vi "GenerateScanEndPts.vi"(0 "X Start":sgl, 1 "Mode":enum16{"Raster", "Serpentine"}(ring), 2 "Calibration In":cluster{dbl, "MicrostepMode":u32}[](array[cluster]), 5 "X End":sgl=9.0, 7 "Y Start":sgl, 9 "Y End":sgl=10.0, 11 "error in":errorcluster, 12 "Line Count":u64=6, 13 "Pixel Count":u64=6, 14 "EdgePt/nPixelMap":bool) -> (4 "Coordinate Array":sgl[][](array[numeric]), 6 "X Pixel Count":u64, 8 "Step Sizes":sgl[](array[numeric]), 10 "Y Pixel Count":u64, 15 "error out":errorcluster)   [LabVIEW 2020]
panel:
  out "Pixel Map":cluster{dbl[], dbl[]}(graph)
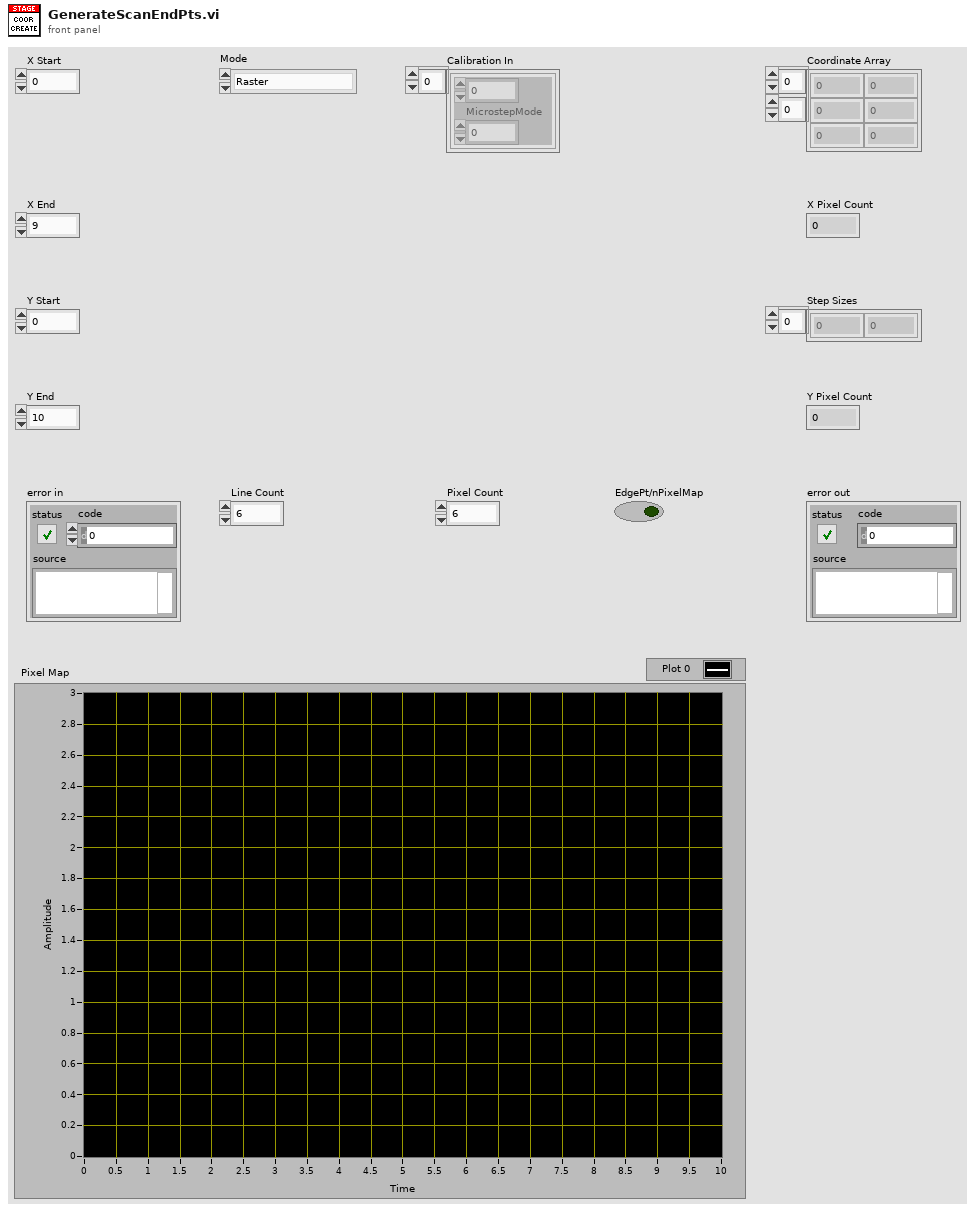
[diagram p1: front panel]
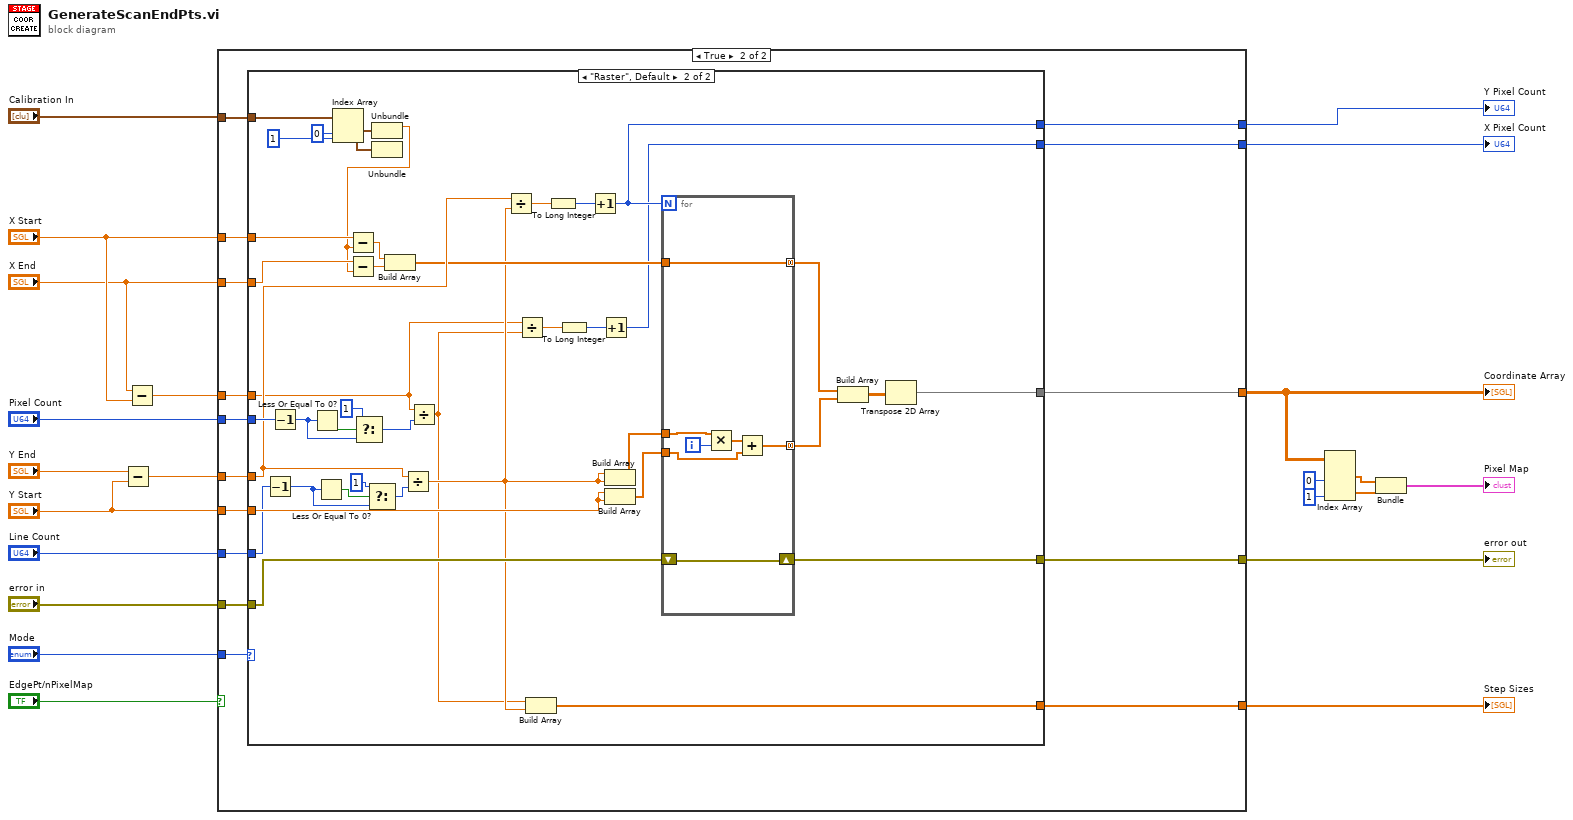
[diagram p0: block diagram]
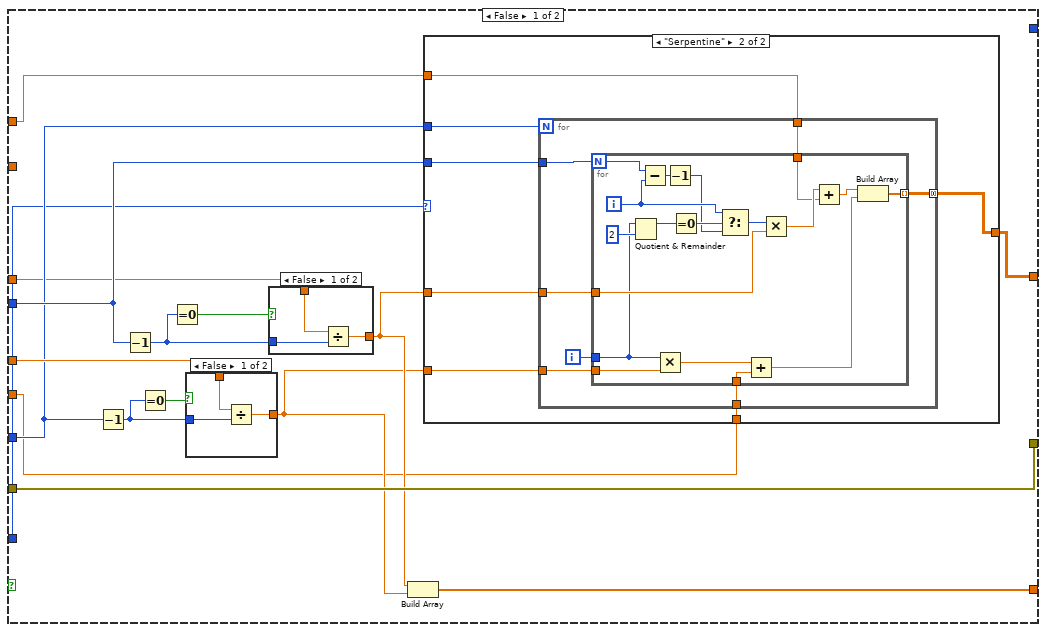
[diagram p2: hidden frame]
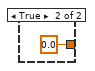
[diagram p3: hidden frame]
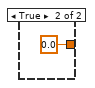
[diagram p4: hidden frame]
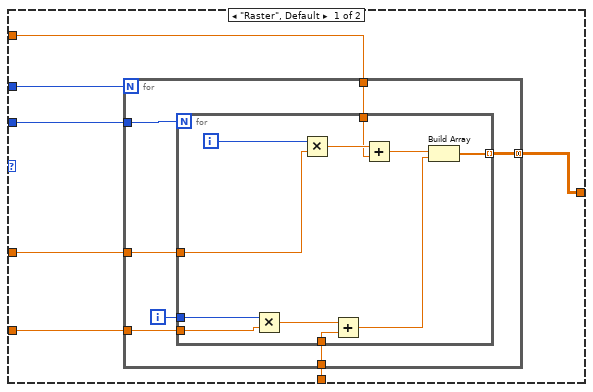
[diagram p5: hidden frame]
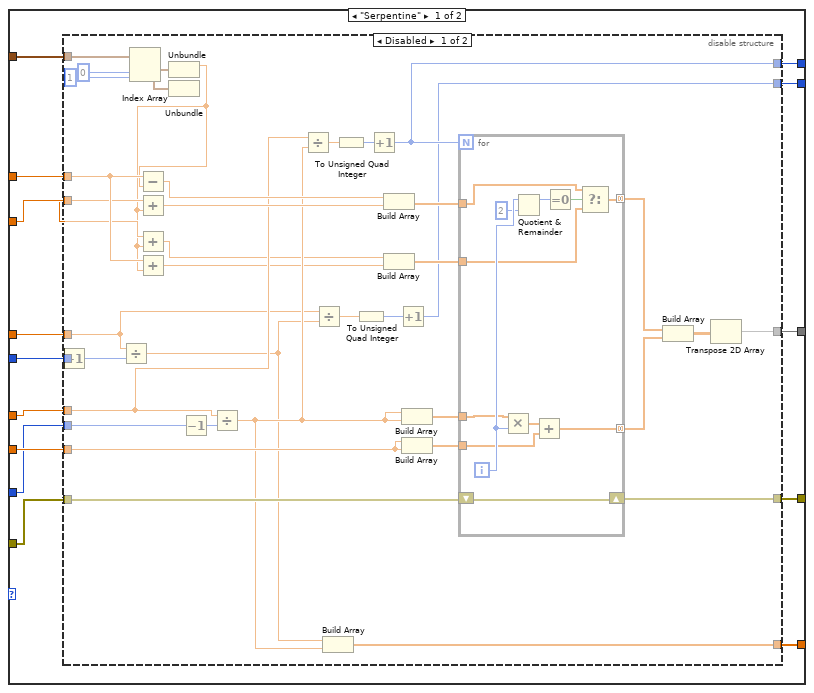
[diagram p6: hidden frame]
diagram:
  n1 = Subtract(x="Y End", y="Y Start") -> (x-y=w20:sgl)
  n2 = Subtract(x="X End", y="X Start") -> (x-y=w16:sgl)
  n3 = case shown="True" "EdgePt/nPixelMap" {
    tunnel: "Y Start" -> [w27 w118]
    tunnel: w20 -> [w36 w110]
    tunnel: "Mode" -> [w29 w106]
    tunnel: "error in" -> [w38 w117]
    tunnel: [w38 w116] -> w17
    tunnel: [w34 w115] -> w3
    tunnel: w16 -> [w30 w114]
    tunnel: "Pixel Count" -> [w37 w111]
    tunnel: "X Start" -> [w28 w107]
    tunnel: [w31 w113] -> w13
    tunnel: "Line Count" -> [w35 w109]
    tunnel: "Calibration In" -> [_ w112]
    tunnel: "X End" -> [_ w108]
    tunnel: [_ w105] -> w2
    tunnel: [_ w104] -> w1
    frame False {
      n4 = Decrement(x=w35) -> (x-1=w26:u64)
      n5 = Decrement(x=w37) -> (x-1=w23:u64)
      n6 = Equal To 0?(x=w26) -> (x = 0?=w25:bool)
      n7 = Equal To 0?(x=w23) -> (x = 0?=w24:bool)
      n8 = case shown="False" w25 {
        tunnel: w36 -> [w45 _]
        tunnel: [w44 sgl 0.0] -> w32
        tunnel: w26 -> [w43 _]
        frame False {
          n9 = Divide(x=w45, y=w43) -> (x/y=w44:sgl)
        }
        frame True {
        }
      }
      n10 = case shown="False" w24 {
        tunnel: [w41 sgl 0.0] -> w33
        tunnel: w30 -> [w40 _]
        tunnel: w23 -> [w39 _]
        frame False {
          n11 = Divide(x=w40, y=w39) -> (x/y=w41:sgl)
        }
        frame True {
        }
      }
      n12 = Build Array(w33, w32) -> (w31:sgl[])
      n13 = case shown="\"Serpentine\"" w29 {
        tunnel: w37 -> [w53 w78]
        tunnel: w35 -> [w52 w77]
        tunnel: [w51 w76] -> w34
        tunnel: w33 -> [w50 w75]
        tunnel: w32 -> [w49 w74]
        tunnel: w28 -> [w48 w73]
        tunnel: w27 -> [w47 w72]
        frame "Raster", Default {
          n14 = for {
            N: w52 -> [_]
            tunnel: w53 -> [w60]
            tunnel: [w59] -> w51 mode=concatenating
            tunnel: w50 -> [w57]
            tunnel: w49 -> [w56]
            tunnel: w48 -> [w55]
            tunnel: w47 -> [w54]
            i -> [w58]
            n15 = for {
              N: w60 -> [_]
              tunnel: [w71] -> w59 mode=indexing
              tunnel: w58 -> [w69]
              tunnel: w57 -> [w67]
              tunnel: w56 -> [w65]
              tunnel: w55 -> [w63]
              tunnel: w54 -> [w61]
              i -> [w70]
              n16 = Multiply(x=w69, y=w65) -> (x*y=w66:sgl)
              n17 = Multiply(x=w70, y=w67) -> (x*y=w68:sgl)
              n18 = Add(x=w66, y=w61) -> (x+y=w62:sgl)
              n19 = Add(x=w68, y=w63) -> (x+y=w64:sgl)
              n20 = Build Array(w64, w62) -> (w71:sgl[])
            }
          }
        }
        frame "Serpentine" {
          n21 = for {
            N: w77 -> [_]
            tunnel: w78 -> [w85]
            tunnel: [w84] -> w76 mode=concatenating
            tunnel: w75 -> [w82]
            tunnel: w74 -> [w81]
            tunnel: w73 -> [w80]
            tunnel: w72 -> [w79]
            i -> [w83]
            n22 = for {
              N: w85 -> [w93]
              tunnel: [w103] -> w84 mode=indexing
              tunnel: w83 -> [w95]
              tunnel: w82 -> [w101]
              tunnel: w81 -> [w99]
              tunnel: w80 -> [w88]
              tunnel: w79 -> [w86]
              i -> [w92]
              n23 = Quotient & Remainder(x=w95, y=2) -> (x-y*floor(x/y)=w96:i32)  [unwired: 1 out]
              n24 = Subtract(x=w93, y=w92) -> (x-y=w91:i32)
              n25 = Multiply(x=w95, y=w99) -> (x*y=w100:sgl)
              n26 = Decrement(x=w91) -> (x-1=w90:i32)
              n27 = Equal To 0?(x=w96) -> (x = 0?=w97:bool)
              n28 = Select(t=w92, s=w97, f=w90) -> (s? t:f=w94:i32)
              n29 = Add(x=w100, y=w86) -> (x+y=w87:sgl)
              n30 = Multiply(x=w94, y=w101) -> (x*y=w102:sgl)
              n31 = Add(x=w102, y=w88) -> (x+y=w89:sgl)
              n32 = Build Array(w89, w87) -> (w103:sgl[])
            }
          }
        }
      }
    }
    frame True {
      n33 = case shown="\"Raster\", Default" w106 {
        tunnel: w118 -> [w132 w223]
        tunnel: w117 -> [w131 w218]
        tunnel: [w130 w217] -> w116
        tunnel: [w129 w215] -> w115
        tunnel: w114 -> [w119 w193]
        tunnel: [w128 w214] -> w113
        tunnel: w112 -> [w127 w211]
        tunnel: w111 -> [w126 w207]
        tunnel: w110 -> [w125 w203]
        tunnel: w109 -> [w124 w202]
        tunnel: w108 -> [w122 w201]
        tunnel: w107 -> [w123 w200]
        tunnel: [w121 w196] -> w105
        tunnel: [w120 w191] -> w104
        frame "Serpentine" {
          n34 = disable-structure shown="Disabled" {
            disable-tunnel: w132 -> [w170 _]
            disable-tunnel: w131 -> [w165 _]
            disable-tunnel: [w164 _] -> w130
            disable-tunnel: [w162 _] -> w129
            disable-tunnel: [w161 _] -> w128
            disable-tunnel: w127 -> [w158 _]
            disable-tunnel: w126 -> [w154 _]
            disable-tunnel: w125 -> [w152 _]
            disable-tunnel: w124 -> [w150 _]
            disable-tunnel: w123 -> [w145 _]
            disable-tunnel: w122 -> [w143 _]
            disable-tunnel: [w140 _] -> w121
            disable-tunnel: [w139 _] -> w120
            disable-tunnel: w119 -> [w138 _]
            frame Disabled {
              n35 = Decrement(x=w154) -> (x-1=w149:u64)
              n36 = Divide(x=w138, y=w149) -> (x/y=w137:sgl)
              n37 = Index Array(array=w158, index #1=0 ("index"), index #2=1 ("index")) -> (element #1=w156:cluster{dbl, "MicrostepMode":u32}, element #2=w157:cluster{dbl, "MicrostepMode":u32})
              n38 = Unbundle(w156) -> (w141:dbl)  [unwired: 1 out]
              n39 = Subtract(x=w145, y=w141) -> (x-y=w155:dbl)
              n40 = Add(x=w143, y=w141) -> (x+y=w153:dbl)
              n41 = Add(x=w143, y=w141) -> (x+y=w142:dbl)
              n42 = Add(x=w145, y=w141) -> (x+y=w144:dbl)
              n43 = Unbundle(w157) -> ()  [unwired: 2 out]
              n44 = Decrement(x=w150) -> (x-1=w148:u64)
              n45 = Divide(x=w152, y=w148) -> (x/y=w151:sgl)
              n46 = Divide(x=w152, y=w151) -> (x/y=w136:sgl)
              n47 = Divide(x=w138, y=w137) -> (x/y=w135:sgl)
              n48 = Build Array(w137, w151) -> (w161:sgl[])
              n49 = To Unsigned Quad Integer(1:w136) -> (0:w133:u64)
              n50 = To Unsigned Quad Integer(1:w135) -> (0:w134:u64)
              n51 = Increment(x=w133) -> (x+1=w140:u64)
              n52 = Build Array(w155, w153) -> (w147:dbl[])
              n53 = Build Array(w142, w144) -> (w146:dbl[])
              n54 = Increment(x=w134) -> (x+1=w139:u64)
              n55 = Build Array(w151, w151) -> (w169:sgl[])
              n56 = Build Array(w170, w170) -> (w168:sgl[])
              n57 = for {
                N: w140 -> [_]
                tunnel: w147 -> [w182]
                tunnel: [w181] -> w167 mode=concatenating
                tunnel: [w178] -> w166 mode=concatenating
                tunnel: w169 -> [w177]
                tunnel: w168 -> [w176]
                tunnel: w146 -> [w171]
                shift-right: [w175] -> w164
                shift-left: w165 -> [w175]
                i -> [w179]
                n58 = Multiply(x=w177, y=w179) -> (x*y=w180:sgl[])
                n59 = Quotient & Remainder(x=w179, y=2) -> (x-y*floor(x/y)=w173:i32)  [unwired: 1 out]
                n60 = Add(x=w180, y=w176) -> (x+y=w178:sgl[])
                n61 = Equal To 0?(x=w173) -> (x = 0?=w172:bool)
                n62 = Select(t=w182, s=w172, f=w171) -> (s? t:f=w181:dbl[])
              }
              n63 = Build Array(w167, w166) -> (w163:dbl[][])
              n64 = Transpose 2D Array(2D array=w163) -> (transposed array=w162:dbl[][])
            }
            frame Enabled {
            }
          }
        }
        frame "Raster", Default {
          n65 = Decrement(x=w202) -> (x-1=w185:u64)
          n66 = Decrement(x=w207) -> (x-1=w188:u64)
          n67 = Less Or Equal To 0?(x=w188) -> (x <= 0?=w189:bool)
          n68 = Less Or Equal To 0?(x=w185) -> (x <= 0?=w184:bool)
          n69 = Index Array(array=w211, index #1=0 ("index"), index #2=1 ("index")) -> (element #1=w209:cluster{dbl, "MicrostepMode":u32}, element #2=w210:cluster{dbl, "MicrostepMode":u32})
          n70 = Select(t=u64 1, s=w189, f=w188) -> (s? t:f=w190:u64)
          n71 = Select(t=u64 1, s=w184, f=w185) -> (s? t:f=w186:u64)
          n72 = Unbundle(w209) -> (w199:dbl)  [unwired: 1 out]
          n73 = Subtract(x=w200, y=w199) -> (x-y=w208:dbl)
          n74 = Subtract(x=w201, y=w199) -> (x-y=w206:dbl)
          n75 = Unbundle(w210) -> ()  [unwired: 2 out]
          n76 = Build Array(w208, w206) -> (w198:dbl[])
          n77 = Divide(x=w203, y=w186) -> (x/y=w197:sgl)
          n78 = Divide(x=w193, y=w190) -> (x/y=w192:sgl)
          n79 = Divide(x=w203, y=w197) -> (x/y=w204:sgl)
          n80 = Divide(x=w193, y=w192) -> (x/y=w194:sgl)
          n81 = Build Array(w192, w197) -> (w214:sgl[])
          n82 = To Long Integer(number=w204) -> (32bit integer=w205:i32)
          n83 = To Long Integer(number=w194) -> (32bit integer=w195:i32)
          n84 = Increment(x=w205) -> (x+1=w196:i32)
          n85 = Increment(x=w195) -> (x+1=w191:i32)
          n86 = Build Array(w197, w197) -> (w222:sgl[])
          n87 = Build Array(w223, w223) -> (w221:sgl[])
          n88 = for {
            N: w196 -> [_]
            tunnel: w198 -> [w230]
            tunnel: [w230] -> w220 mode=concatenating
            tunnel: [w227] -> w219 mode=concatenating
            tunnel: w222 -> [w226]
            tunnel: w221 -> [w225]
            shift-right: [w224] -> w217
            shift-left: w218 -> [w224]
            i -> [w228]
            n89 = Multiply(x=w226, y=w228) -> (x*y=w229:sgl[])
            n90 = Add(x=w229, y=w225) -> (x+y=w227:sgl[])
          }
          n91 = Build Array(w220, w219) -> (w216:dbl[][])
          n92 = Transpose 2D Array(2D array=w216) -> (transposed array=w215:dbl[][])
        }
      }
    }
  }
  "Coordinate Array" <- w3
  "error out" <- w17
  "Step Sizes" <- w13
  "Y Pixel Count" <- w2
  "X Pixel Count" <- w1
  n93 = Index Array(array=w3, index (col) #1=0 ("disabled index (col)"), index (col) #2=1 ("index (col)")) -> (element #1=w6:dbl[], element #2=w5:dbl[])  [unwired: 2 in]
  n94 = Bundle(w6, w5) -> (→"Pixel Map":cluster{dbl[], dbl[]})  [unwired: 1 in]
